vi "SiosIfmI2CWrite.vi"(0 "Device Number":i32, 1 "i2c Addres":i32, 2 "RAM Addres":i32, 3 "count":i32, 4 "Buffer":string) -> (5 "success":i32)   [LabVIEW 2009]
uses:
  siosifm.dll
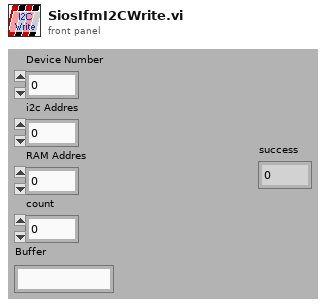
[diagram p1: front panel]
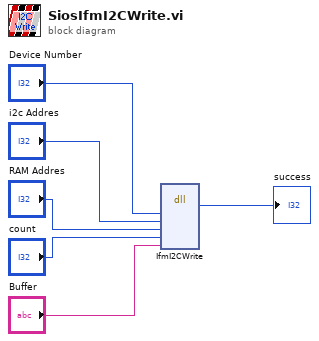
[diagram p0: block diagram]
diagram:
  n1 = dll-call lib="C:/WORK/Artem/RE-10/SIOS_IfmDLL/siosifm.dll" fn="IfmI2CWrite"("devNumber"="Device Number", "i2c_addr"="i2c Addres", "ram_addr"="RAM Addres", "count"="count", "buffer"="Buffer") -> ("success"=→"success":i32)  [unwired: 8 in, 2 out]
